vi "9474PWM.vi"() -> ()   [LabVIEW 2013]
panel:
  in  "Boolean":bool
  out "error out":errorcluster
  in  "stop":bool
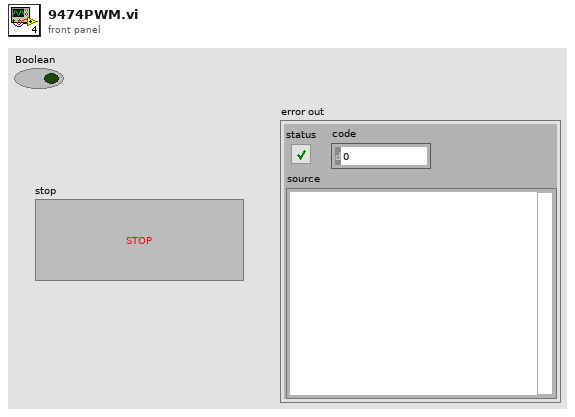
[diagram p1: front panel]
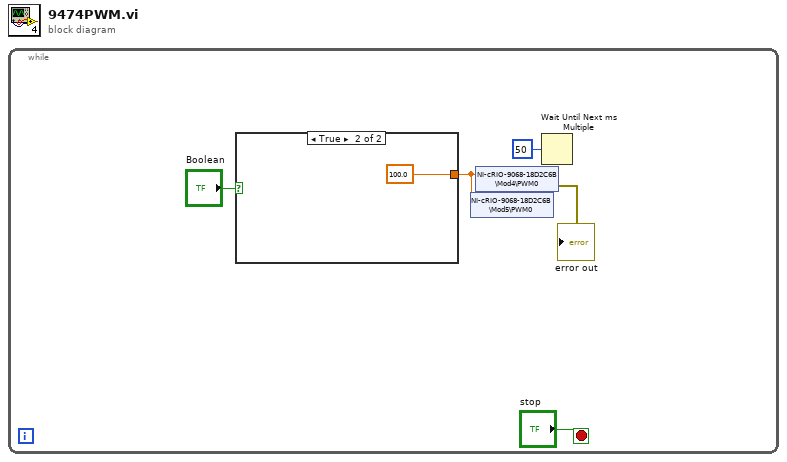
[diagram p0: block diagram]
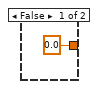
[diagram p2: hidden frame]
diagram:
  n1 = while {
    stop <- "stop" stop-if-true
    n2 = case shown="True" "Boolean" {
      tunnel: [0.0 ("PWM0") 100.0 ("PWM0")] -> w3
      frame False {
      }
      frame True {
      }
    }
    n3 = shared-variable "NI-cRIO-9068-18D2C6B\\Mod5\\PWM0"(w3) -> ()  [unwired: 1 in, 1 out]
    n4 = shared-variable "NI-cRIO-9068-18D2C6B\\Mod4\\PWM0"(w3) -> (error out=→"error out":errorcluster)  [unwired: 1 in]
    n5 = Wait Until Next ms Multiple(millisecond multiple=u32 50) -> ()  [unwired: 1 out]
  }
